vi "DSF.Engine.Plugin.Transfer Group.Send.vi"(7 "Command":T1=enum."Tx", 8 "error in (no error)":errorcluster, 10 "Transfer Group in":refnum<class "DSF.Engine.Transfer Group.lvclass">, 11 "Plugin in":refnum<class "DSF.Engine.Plugin.lvclass">) -> (0 "error out":errorcluster, 2 "Transfer Group out":refnum<class "DSF.Engine.Transfer Group.lvclass">, 3 "Plugin out":refnum<class "DSF.Engine.Plugin.lvclass">)   [LabVIEW 2017, in "DSF.Engine.lvlib" / "DSF.Engine.Plugin.lvclass"]
uses:
  DSF.Engine.Plugin.lvclass
  Transfer/DSF.Engine.Transfer Group.lvclass
  Interface/DSF.Engine.Interface.Transceiver.Command.ctl
  Interface/DSF.Engine.Interface.Transceiver.lvclass
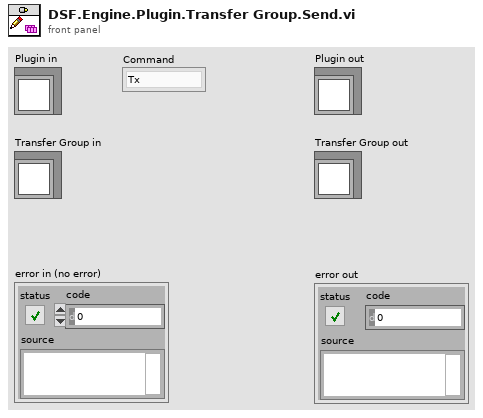
[diagram p1: front panel]
types:
  T1 = typedef "DSF.Engine.lvlib/DSF.Engine.Interface.Transceiver.lvclass/DSF.Engine.Interface.Transceiver.Command.ctl" = enum8{"Rx", "Tx", "Shutdown"}
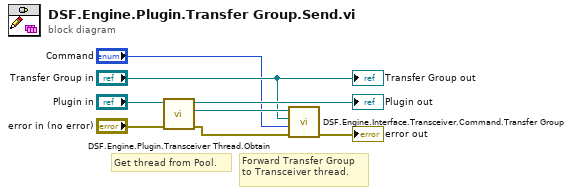
[diagram p0: block diagram]
diagram:
  # "Forward Transfer Group to Transceiver thread."
  # "Get thread from Pool."
  n1 = call "DSF.Engine.Plugin.Transceiver Thread.Obtain.vi"("error in (no error)"="error in (no error)", "Plugin in"="Plugin in") -> ("error out"=w6:errorcluster, "Transceiver Thread"=w7:refnum<class "DSF.Engine.Interface.Transceiver.lvclass">, "Plugin out"=→"Plugin out":refnum<class "DSF.Engine.Plugin.lvclass">)  [unwired: 7 in]
  n2 = call "DSF.Engine.Interface.Transceiver.Command.Transfer Group.vi"("error in (no error)"=w6, "Command"="Command", "Transfer Group"="Transfer Group in", "Transceiver Interface in"=w7) -> ("error out"=→"error out":errorcluster)  [unwired: 6 in, 1 out]
  "Transfer Group out" <- "Transfer Group in"
